vi "Get Attribute Tree Data.vi"(7 "Tree ID":string, 8 "Error In":errorcluster, 10 "Attribute Name":string, 11 "Tree Manager":T1) -> (0 "Error Out":errorcluster, 1 "Attribute Value":refnum<class "Tree Data.lvclass">, 2 "Found?":bool, 3 "Tree Manager":T1)   [LabVIEW 2020, in "NI_VIAnCFGDataStructure.lvlib" / "Tree.lvclass"]
doc: "Get a Tree Data attribute of the Tree."
uses:
  <vilib>/addons/analyzer/VIAnCFGDataStructure/Tree Manager/Tree.lvclass
  <vilib>/addons/analyzer/VIAnCFGDataStructure/Tree Manager/Typedefs/Session Handle.ctl
  <vilib>/addons/analyzer/VIAnCFGDataStructure/Tree Data/Tree Data.lvclass
  <vilib>/addons/analyzer/VIAnCFGDataStructure/Tree Manager/Tree.lvclass/Tree.ctl
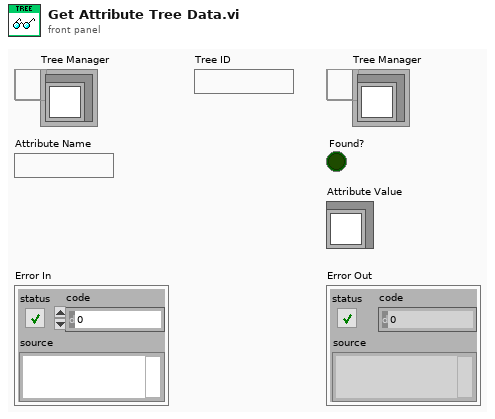
[diagram p1: front panel]
types:
  T1 = typedef "NI_VIAnCFGDataStructure.lvlib/Tree.lvclass/Session Handle.ctl" = refnum<data-value>
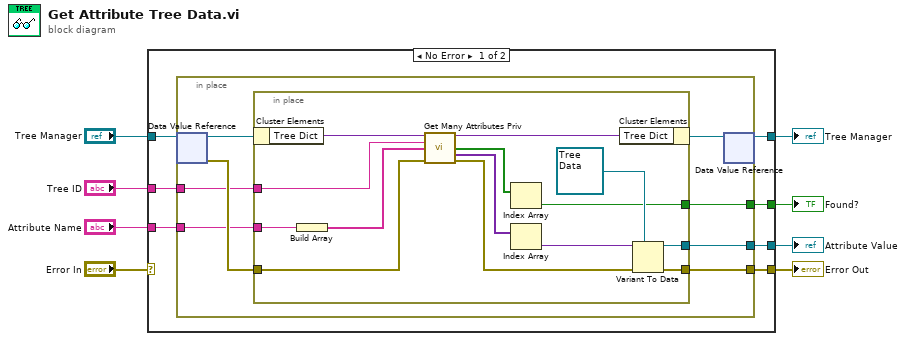
[diagram p0: block diagram]
diagram:
  n1 = case shown="No Error" "Error In" {
    selector: "Error In" -> [_ w38]
    tunnel: "Tree Manager" -> [w15 w39]
    tunnel: [w14 w39] -> w7
    tunnel: [w13 w38] -> w5
    tunnel: "Tree ID" -> [w12 _]
    tunnel: "Attribute Name" -> [w11 _]
    tunnel: [w10 _] -> w2
    tunnel: [w9 _] -> w1
    frame No Error {
      n2 = in-place {
        in-place-border: [w22] -> w13
        in-place-border: w12 -> [w19]
        in-place-border: w11 -> [w18]
        in-place-border: [w17] -> w10
        in-place-border: [w16] -> w9
        n3 = in-place-dvr #1(w15) -> (w23:refnum<class "Tree.lvclass">, w20:errorcluster)
        n4 = in-place {
          in-place-border: [w37] -> w22
          in-place-border: w20 -> [w29]
          in-place-border: w19 -> [w32]
          in-place-border: w18 -> [w31]
          in-place-border: [w26] -> w17
          in-place-border: [w35] -> w16
          n5 = in-place-cluster #2(w23) -> ("Tree Dict"=w34:variant)
          n6 = Build Array(w31) -> (w30:string[])
          n7 = call <vilib>:"Get Many Attributes Priv.vi"("Tree Dictionary In"=w34, "Unique ID"=w32, "Attribute Names"=w30, "error in"=w29) -> ("Tree Dictionary Out"=w33:variant, "Found?"=w27:bool[], "Attribute Values"=w25:variant[], "error out"=w28:errorcluster)  [unwired: 7 in, 1 out]
          n8 = Index Array(array=w27) -> (element=w26:bool)  [unwired: 1 in]
          n9 = Index Array(array=w25) -> (element=w24:variant)  [unwired: 1 in]
          n10 = in-place-cluster #2("Tree Dict"=w33) -> (w21:refnum<class "Tree.lvclass">)
          n11 = Variant To Data(error in=w28, type=refnum<class "Tree Data.lvclass"> refnum ("Tree Data.lvclass"), Variant=w24) -> (data=w35:refnum<class "Tree Data.lvclass">, error out=w37:errorcluster)
        }
        n12 = in-place-dvr #1(w21) -> (w14:T1)  [unwired: 1 out]
      }
    }
    frame Error {
    }
  }
  "Tree Manager" <- w7
  "Error Out" <- w5
  "Found?" <- w2
  "Attribute Value" <- w1
